vi "MT Generate PSK Synchronization Parameters (number array).vi"(0 "PSK system parameters":T1={"samples per symbol (16)"=16, "symbol map"=[], "differential PSK"=enum."disable", "PSK type"=0} {"PSK type" items=["normal", "shifted", "offset"]; "symbol map" format="%.3f"}, 5 "sync numbers":i32[](array[numeric]) format="%.0x", 7 "bits per sync number":i32=32, 11 "error in (no error)":errorcluster, 12 "expected sync location (symbols)":i32=-1, 13 "sync location uncertainty (symbols)":i32=10, 14 "sync indent (symbols)":i32) -> (4 "PSK synchronization parameters":T2 {"sync sequence" format="%.2f"}, 15 "error out":errorcluster)   [LabVIEW 2020, in "niDMT.lvlib"]
doc: "This polymorphic instance generates synchronization parameters for PSK demodulation using a synchronization sequence defined by a <B>sync numbers</B> array in which each number represents a group of bits."
uses:
  <vilib>/addons/Modulation/niDMT.lvlib
  <vilib>/addons/Modulation/niAMT.lvlib
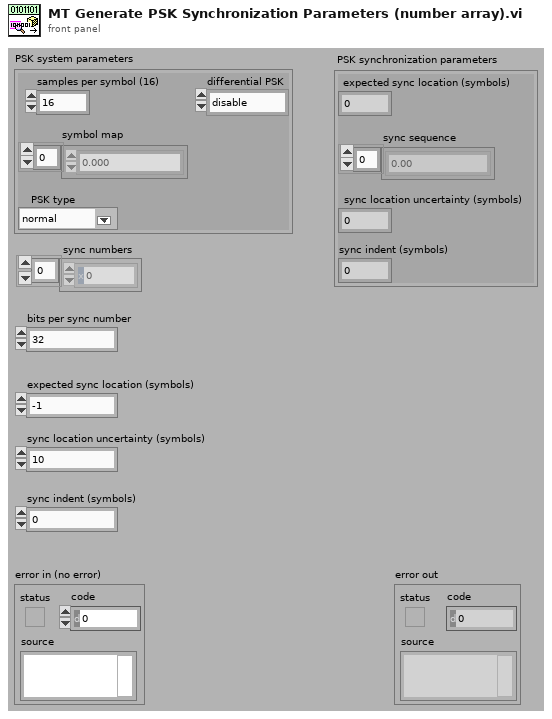
[diagram p1: front panel]
types:
  T1 = cluster{"samples per symbol (16)":i32, "symbol map":cdb[], "differential PSK":enum16{"disable", "enable"}, "PSK type":u16}
  T2 = cluster{"expected sync location (symbols)":i32, "sync sequence":cdb[], "sync location uncertainty (symbols)":i32, "sync indent (symbols)":i32}
  T3 = typedef "niDMT.lvlib/PSK Sync Parameters.ctl" = cluster{"expected sync location (symbols)":i32, "sync sequence":cdb[], "sync location uncertainty (symbols)":i32, "sync indent (symbols)":i32}
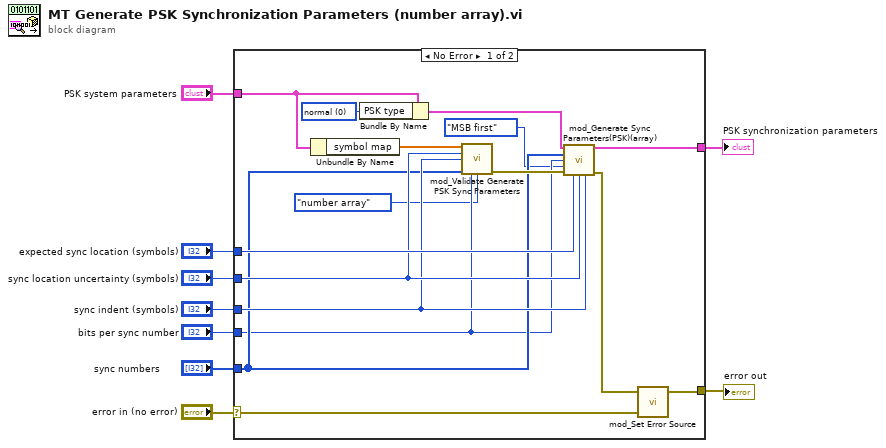
[diagram p0: block diagram]
diagram:
  n1 = case shown="No Error" "error in (no error)" {
    selector: "error in (no error)" -> [w24 w26]
    tunnel: "expected sync location (symbols)" -> [w23 _]
    tunnel: "sync location uncertainty (symbols)" -> [w18 _]
    tunnel: "sync indent (symbols)" -> [w17 _]
    tunnel: "sync numbers" -> [w16 _]
    tunnel: "bits per sync number" -> [w15 _]
    tunnel: [w25 w26] -> w3
    tunnel: "PSK system parameters" -> [w12 _]
    tunnel: [w22 _] -> w1
    frame No Error {
      w10 = u16 0 items=["normal", "shifted", "offset"] ("PSK type")
      n2 = Unbundle By Name(w12) -> ("symbol map"=w19:cdb[])
      n3 = Bundle By Name(cluster=w12, "PSK type"=w10) -> (w11:T1)
      n4 = call <vilib>:"mod_Validate Generate PSK Sync Parameters.vi"("symbol map"=w19, "sync location uncertainty (symbols)"=w18, "sync indent (symbols)"=w17, "sync numbers"=w16, "number of bits (or) bits per number"=w15, "sync bits specification"=enum16{"bit array", "number array", "number"}."number array") -> ("error out"=w20:errorcluster)  [unwired: 1 in, 8 out]
      n5 = call <vilib>:"mod_Generate Sync Parameters(PSK)(array).vi"("PSK system parameters"=w11, "sync numbers"=w16, "bits per number"=w15, "bit order"=enum16{"MSB first", "LSB first"}."MSB first", "error in (no error)"=w20, "expected sync location (symbols)"=w23, "sync location uncertainty (symbols)"=w18, "sync indent (symbols)"=w17) -> ("PSK synchronization parameters"=w22:T3, "error out"=w21:errorcluster)  [unwired: 6 out]
      n6 = call <vilib>:"mod_Set Error Source.vi"("initial error in (no error)"=w24, "final error in (no error)"=w21) -> ("error out"=w25:errorcluster)  [unwired: 3 out]
    }
    frame Error {
    }
  }
  "PSK synchronization parameters" <- w1
  "error out" <- w3
